vi "2D Linear Evaluation (CDB).vi"(2 "b":cdb format="%#.2g", 3 "a":cdb format="%#.2g", 4 "X":cdb[][](array[numeric])) -> (0 "error":i32, 1 "Y[i,j]=X[i,j]*a+b":cdb[][](array[numeric]))   [LabVIEW 2018, in "NI_AALPro.lvlib"]
doc: "Performs a linear evaluation on every element of <B>X</B> using the scale <B>a</B> and the offset <B>b</B>. Wire data to the <B>X</B> input to determine the polymorphic instance to use or manually select the instance."
uses:
  NI_AALPro.lvlib
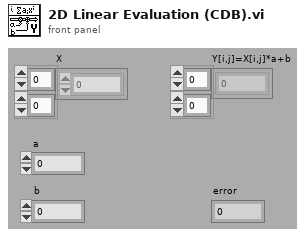
[diagram p1: front panel]
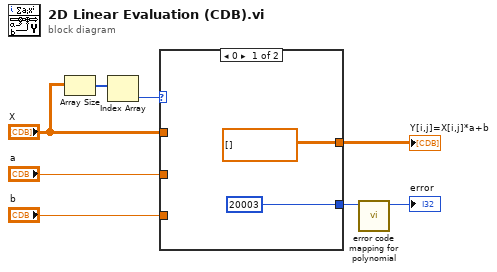
[diagram p0: block diagram]
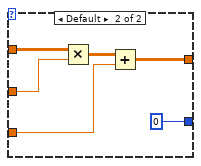
[diagram p2: hidden frame]
diagram:
  n1 = Array Size(array="X") -> (size(s)=w8:i32[])
  n2 = Index Array(array=w8) -> (element=w7:i32)  [unwired: 1 in]
  n3 = case shown="0" w7 {
    tunnel: "X" -> [_ w16]
    tunnel: "a" -> [_ w15]
    tunnel: "b" -> [_ w13]
    tunnel: [cdb[][] [] w12] -> w3
    tunnel: [20003 ("empty array") 0] -> w2
    frame 0 {
    }
    frame Default {
      n4 = Multiply(x=w16, y=w15) -> (x*y=w14:cdb[][])
      n5 = Add(x=w14, y=w13) -> (x+y=w12:cdb[][])
    }
  }
  "Y[i,j]=X[i,j]*a+b" <- w3
  n6 = call "error code mapping for polynomial.vi"("error in"=w2) -> ("error out"=→"error":i32)  [unwired: 10 in]
